vi "XML ( Delete Node Value Multiple Inputs ).vi"(8 "error in (no error)":errorcluster, 9 "Child_Node":string[](array[string]), 10 "Parent_Node":string[](array[string]), 11 "XML in":refnum<class "XML.lvclass">) -> (0 "error out":errorcluster, 3 "XML out":refnum<class "XML.lvclass">)   [LabVIEW 2018, in "XML.lvlib" / "XML.lvclass"]
uses:
  XML.lvclass
  XML.lvclass/XML.ctl
  <vilib>/xml/Close Reference(Node).vi
  <vilib>/xml/NI_XML.lvlib
  <resource>/objmgr/DOMUserDefRef.rc
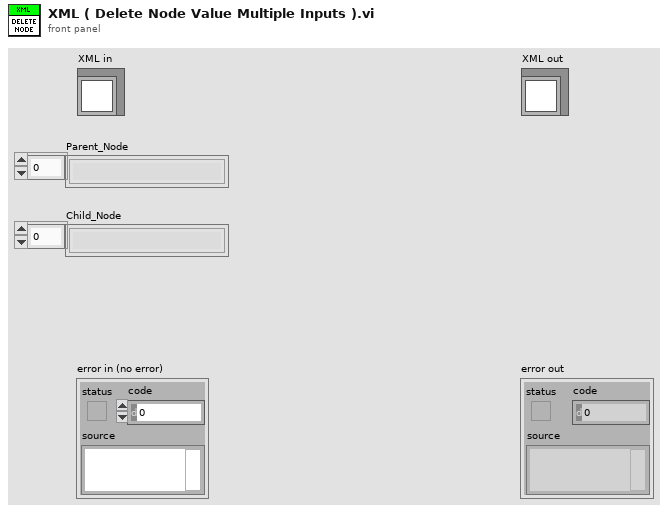
[diagram p1: front panel]
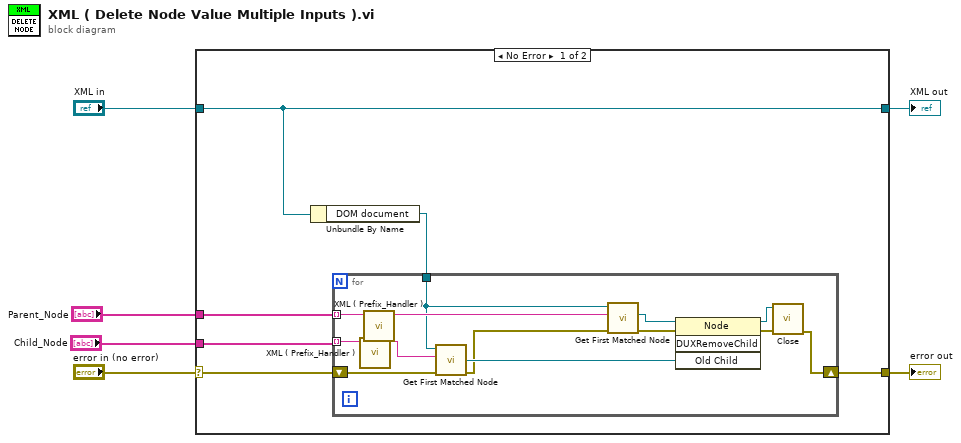
[diagram p0: block diagram]
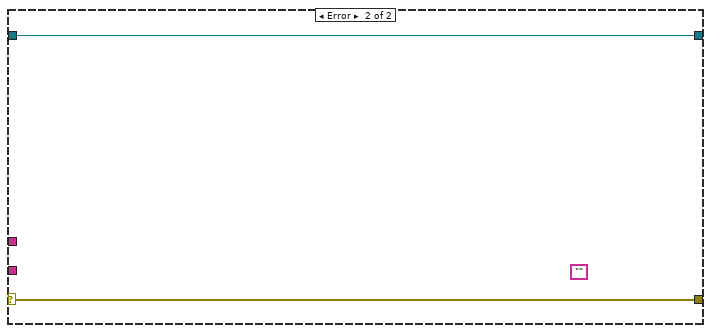
[diagram p2: hidden frame]
diagram:
  n1 = case shown="No Error" "error in (no error)" {
    selector: "error in (no error)" -> [w7 w27]
    tunnel: [w11 w27] -> w5
    tunnel: [w12 w26] -> w3
    tunnel: "XML in" -> [w12 w26]
    tunnel: "Parent_Node" -> [w10 _]
    tunnel: "Child_Node" -> [w9 _]
    frame No Error {
      n2 = Unbundle By Name(w12) -> ("DOM document"=w8:refnum<k20>)
      n3 = for {
        tunnel: w10 -> [w20] mode=indexing
        tunnel: w9 -> [w18] mode=indexing
        tunnel: w8 -> [w17]
        shift-right: [w21] -> w11
        shift-left: w7 -> [w15]
        n4 = call "XML ( Prefix_Handler ).vi"("input string"=w18) -> ("result string"=w16:string)  [unwired: 10 in]
        n5 = call "XML ( Prefix_Handler ).vi"("input string"=w20) -> ("result string"=w19:string)  [unwired: 10 in]
        n6 = call <vilib>:"Get First Matched Node.vi"("error in (no error)"=w15, "XPath expression"=w16, "node in"=w17) -> ("error out"=w13:errorcluster, "node result"=w14:refnum<k20>)  [unwired: 6 in, 1 out]
        n7 = call <vilib>:"Get First Matched Node.vi"("error in (no error)"=w13, "XPath expression"=w19, "node in"=w17) -> ("error out"=w24:errorcluster, "node result"=w25:refnum<k20>)  [unwired: 6 in, 1 out]
        n8 = invoke class="Node" method="DUXRemoveChild"(reference=w25, error in=w24, "Old Child"=w14) -> (reference out=w22:refnum<k20>, error out=w23:errorcluster)  [unwired: 1 in, 2 out]
        n9 = call-poly <vilib>:"Close.vi"("error in (no error)"=w23, "node"=w22) -> ("error out"=w21:errorcluster)  [unwired: 7 in]
      }
    }
    frame Error {
      (unwired) ""
    }
  }
  "error out" <- w5
  "XML out" <- w3
